vi "Prepare LV to Use Icon Editor Source.vi"   [LabVIEW 2024]
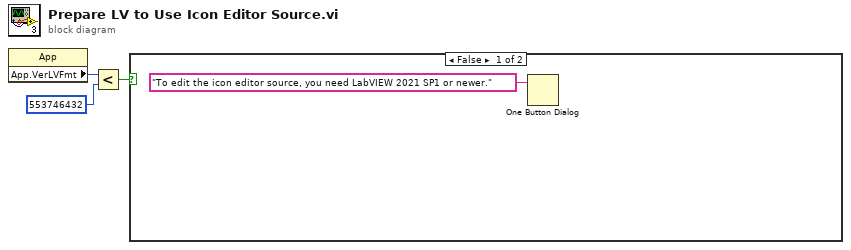
[diagram p0: block diagram]
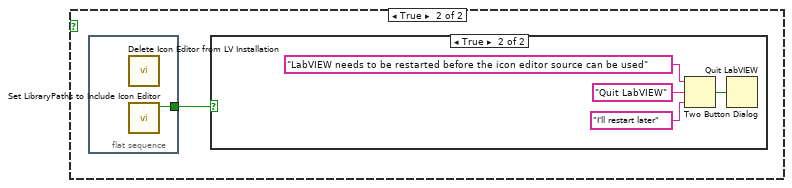
[diagram p2: hidden frame]
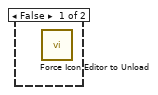
[diagram p3: hidden frame]
diagram:
  n1 = property class="App"() -> ("App.VerLVFmt"=w3:i32)  [unwired: 2 in, 2 out]
  n2 = Less?(x=w3, y=553746432 ("Application:Version As Integer")) -> (x < y?=w1:bool)
  n3 = case shown="False" w1 {
    frame False {
      n4 = One Button Dialog(message="To edit the icon editor source, you need LabVIEW 2021 SP1 or newer.") -> ()  [unwired: 1 in, 1 out]
    }
    frame True {
      n5 = flat-sequence {
        tunnel: [w6] -> w5
        frame #0 {
          n6 = call <resource>:"Delete Icon Editor from LV Installation.vi"() -> ()  [unwired: 10 in, 2 out]
          n7 = call <resource>:"Set LibraryPaths to Include Icon Editor.vi"() -> ("config modified?"=w6:bool)  [unwired: 10 in, 1 out]
        }
      }
      n8 = case shown="True" w5 {
        frame False {
          n9 = call <resource>:"Force Icon Editor to Unload.vi"() -> ()  [unwired: 12 in]
        }
        frame True {
          n10 = Two Button Dialog(message="LabVIEW needs to be restarted before the icon editor source can be used", 1:"I'll restart later" ("F button name (\"Cancel\")"), 2:"Quit LabVIEW" ("T button name (\"OK\")")) -> (T button?=w10:bool)
          n11 = Quit LabVIEW(quit? (T)=w10) -> ()
        }
      }
    }
  }
